vi "RemoveComments.vi"(3 "Via file in":string) -> (1 "Via file out":string)   [LabVIEW 2014]
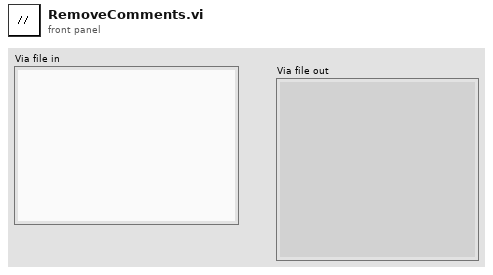
[diagram p1: front panel]
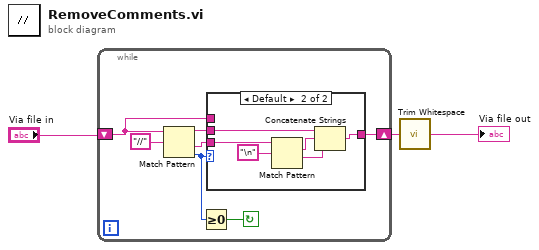
[diagram p0: block diagram]
diagram:
  n1 = while {
    shift-right: [w7] -> w3
    shift-left: "Via file in" -> [w4]
    stop <- w6 continue-if-true
    n2 = Match Pattern(string=w4, regular expression="//") -> (before substring=w8:string, after substring=w9:string, offset past match=w5:i32)  [unwired: 1 in, 1 out]
    n3 = Greater Or Equal To 0?(x=w5) -> (x >= 0?=w6:bool)
    n4 = case shown="Default" w5 {
      tunnel: w9 -> [_ w17]
      tunnel: w8 -> [_ w15]
      tunnel: [w11 w14] -> w7
      tunnel: w4 -> [w11 _]
      frame -1 {
      }
      frame Default {
        n5 = Match Pattern(string=w17, regular expression="\n") -> (match substring=w12:string, after substring=w13:string)  [unwired: 1 in, 2 out]
        n6 = Concatenate Strings(w15, w12, w13) -> (w14:string)
      }
    }
  }
  n7 = call <vilib>:"Trim Whitespace.vi"("string"=w3) -> ("trimmed string"=→"Via file out":string)  [unwired: 1 in]
